vi "Extract LineData.vi"(3 "ROI End":u32, 4 "Input Data":u32[][](array[numeric]), 5 "ROI Beg":u32) -> (0 "no of spectra":i32, 1 "ROI Data":u32[](array[numeric]), 2 "Sum spectra":u32[](graph))   [LabVIEW 2015]
panel:
  out "no of channels":i32
  out "Max Spectra":u32[](graph)
  out "Intensity Graph":u32[][](graph)
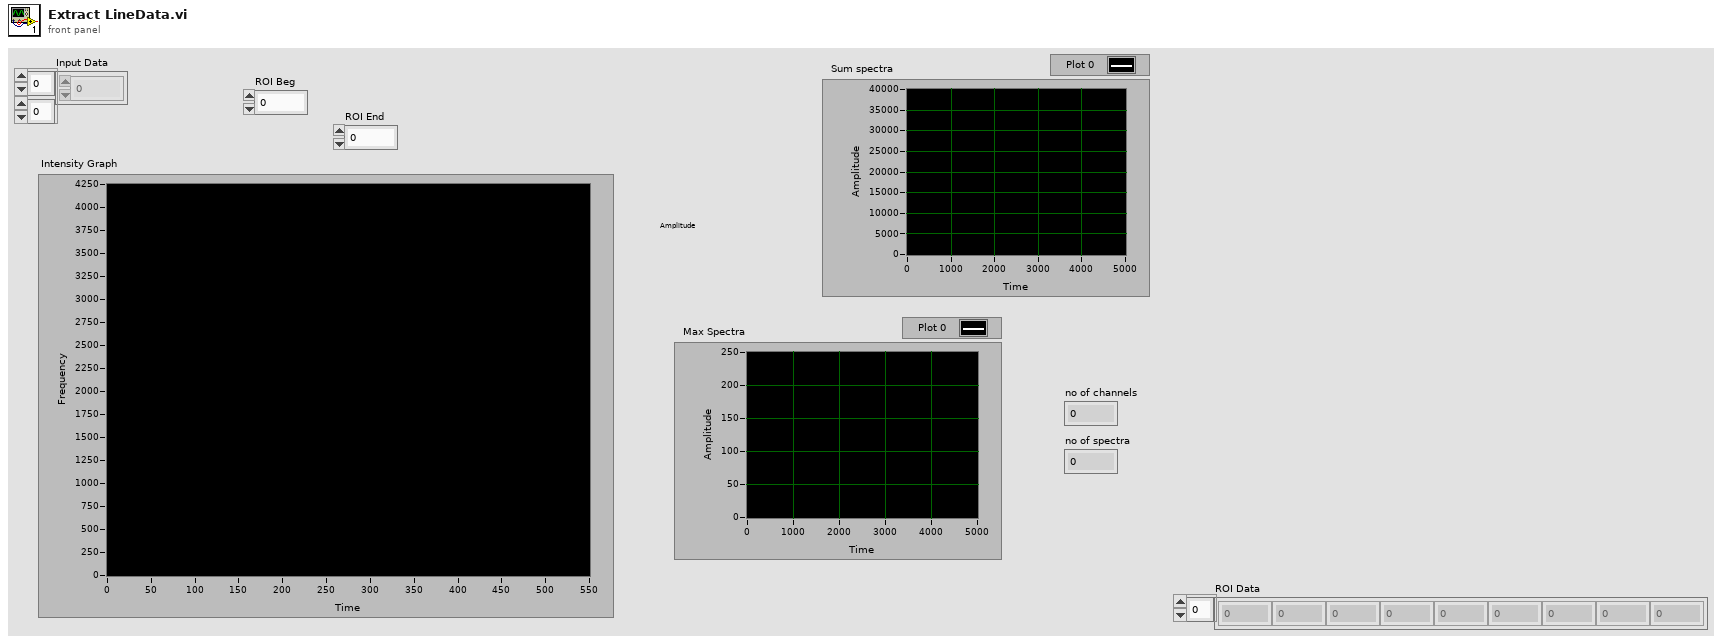
[diagram p1: front panel]
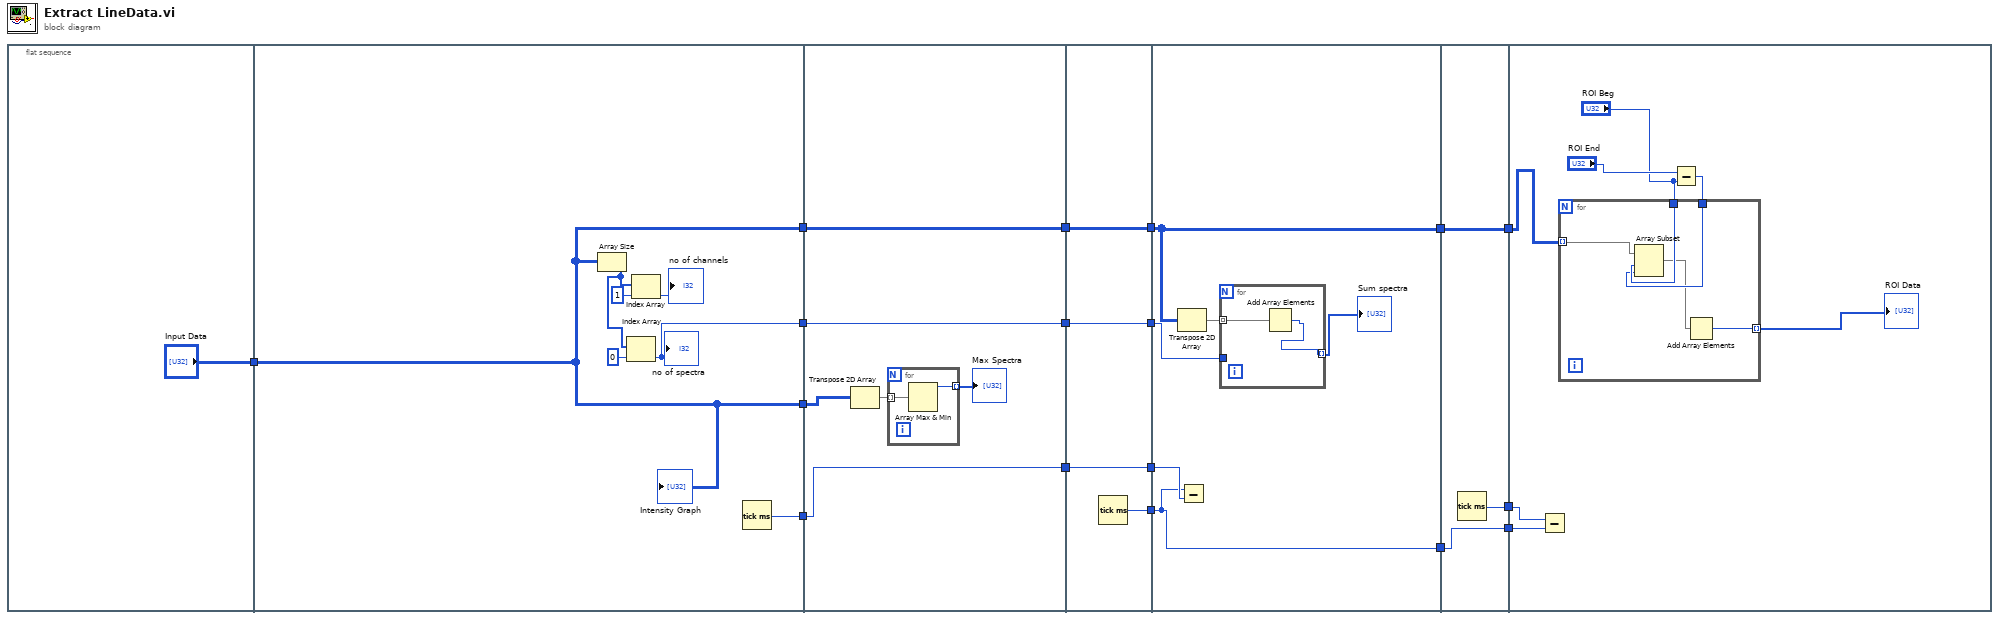
[diagram p0: block diagram]
diagram:
  n1 = flat-sequence {
    tunnel: ["Input Data"] -> w6
    tunnel: [w25] -> w17
    tunnel: [w24] -> w16
    tunnel: [w24] -> w10
    tunnel: w6 -> [w24]
    tunnel: [w19] -> w3
    tunnel: w17 -> [w28]
    tunnel: w16 -> [w31]
    tunnel: [w28] -> w15
    tunnel: [w27] -> w11
    tunnel: w10 -> [w27]
    tunnel: [w26] -> w4
    tunnel: w3 -> [w26]
    tunnel: w15 -> [w37]
    tunnel: [w37] -> w14
    tunnel: [w36] -> w13
    tunnel: [w35] -> w12
    tunnel: w11 -> [w35]
    tunnel: [w34] -> w5
    tunnel: w4 -> [w34]
    tunnel: w14 -> [w43]
    tunnel: w13 -> [w41]
    tunnel: w12 -> [w38]
    tunnel: [w41] -> w9
    tunnel: w5 -> [w40]
    tunnel: [w38] -> w1
    tunnel: w9 -> [w47]
    tunnel: [w48] -> w8
    tunnel: [w47] -> w7
    tunnel: [w46] -> w2
    tunnel: w1 -> [w46]
    tunnel: w8 -> [w55]
    tunnel: w7 -> [w54]
    tunnel: w2 -> [w49]
    frame #0 {
    }
    frame #1 {
      n2 = Array Size(array=w24) -> (size(s)=w20:i32[])
      n3 = Index Array(array=w20, index=0) -> (element=w19:i32)
      "no of spectra" <- w19
      n4 = Index Array(array=w20, index=1) -> (element=→"no of channels":i32)
      n5 = Tick Count (ms)() -> (millisecond timer value=w25:u32)
      "Intensity Graph" <- w24
    }
    frame #2 {
      n6 = Transpose 2D Array(2D array=w31) -> (transposed array=w30:u32[][])
      n7 = for {
        tunnel: w30 -> [w33] mode=indexing
        tunnel: [w32] -> w29 mode=indexing
        n8 = Array Max & Min(array=w33) -> (max value=w32:u32)  [unwired: 3 out]
      }
      "Max Spectra" <- w29
    }
    frame #3 {
      n9 = Tick Count (ms)() -> (millisecond timer value=w36:u32)
    }
    frame #4 {
      n10 = Transpose 2D Array(2D array=w38) -> (transposed array=w42:u32[][])
      n11 = Subtract(x=w41, y=w43) -> ()  [unwired: 1 out]
      n12 = for {
        tunnel: w42 -> [w45] mode=indexing
        tunnel: w40 -> [_]
        tunnel: [w44] -> w39 mode=indexing
        n13 = Add Array Elements(numeric array=w45) -> (sum=w44:u32)
      }
      "Sum spectra" <- w39
    }
    frame #5 {
      n14 = Tick Count (ms)() -> (millisecond timer value=w48:u32)
    }
    frame #6 {
      n15 = Subtract(x=w55, y=w54) -> ()  [unwired: 1 out]
      n16 = Subtract(x="ROI End", y="ROI Beg") -> (x-y=w51:u32)
      n17 = for {
        tunnel: w49 -> [w60] mode=indexing
        tunnel: "ROI Beg" -> [w59]
        tunnel: w51 -> [w58]
        tunnel: [w56] -> w50 mode=indexing
        n18 = Array Subset(array=w60, index=w59, length=w58) -> (w57:u32[])
        n19 = Add Array Elements(numeric array=w57) -> (sum=w56:u32)
      }
      "ROI Data" <- w50
    }
  }
